vi "measure_j-t.vi"(4 "Skip pixel?":bool, 5 "Date array":string[](array[string]), 6 "Scan settings":T1={"J-V scan"=TRUE, "Start voltage (V)"=0.0, "End voltage (V)"=0.0, "Step voltage (V)"=1.4, "Scan both directions"=TRUE, "Inverted device structure"=FALSE, "Measurement delay (ms)"=10.0, "Measurement speed"=0, "Scan rate (V/s)"=0.0, "Stabilisation time (s)"=0.0, "Stabilisation mode"=0, "Stabilisation value (V or A) "=1.0, "Illumination"=0, "Stabilisation in the dark?"=FALSE, "Repeat light scans"=FALSE, "No. of repeat scans"=0.0, "Only repeat for best pixel"=1, "J-t scan"=FALSE, "J-t best pixel only"=7, "J-t start voltage (V)"=0.0, "J-t end voltage (V)"=1.4, "J-t step voltage (V)"=0.01, "Step time (s)"=0.7, "J-t scan both directions"=TRUE, "J-t inverted device structure"=FALSE, "J-t settling delay (s)"=0.0, "J-t measurement speed"=0, "J-t illumination"=2, "Max. power stabilisation"=FALSE, "Max power best pixel only"=1, "Max. power point tracker"=FALSE, "Vmp from J-V scan"=FALSE, "Max P stab. Specific voltage"=FALSE, "Vmp (V)"=1.0, "Stabilisation time step (s)"=1.0, "Total stabilisation time (s)"=100.0} {"J-t settling delay (s)" min=10.0; "J-t illumination" items=["Light only", "Dark only", "Light then dark", "Dark then light"]; "Measurement speed" items=["Fast", "Normal", "High accuracy"]; "Illumination" items=["Light only", "Dark only", "Light then dark", "Dark then light"]; "Only repeat for best pixel" items=["only for best pixel", "for best 2 pixels", "for best 3 pixels", "for best 4 pixels", "for best 5 pixels", "for best 6 pixels", "for best 7 pixels", "for all pixels"]; "No. of repeat scans" min=1.0 step=1.0; "Max power best pixel only" items=["only the best pixel", "the best 2 pixels", "the best 3 pixels", "the best 4 pixels", "the best 5 pixels", "the best 6 pixels", "the best 7 pixels", "all pixels"]; "J-t best pixel only" items=["only the best pixel", "the best 2 pixels", "the best 3 pixels", "the best 4 pixels", "the best 5 pixels", "the best 6 pixels", "the best 7 pixels", "all pixels"]; "J-t measurement speed" items=["Fast", "Normal", "High Accuracy"]; "Stabilisation mode" items=["V", "I"]; "Measurement delay (ms)" min=10.0}, 7 "Cell details cluster":T2={"Cell Position"=16, "Cell Label"="", "Pixel to measure"=0, "Area (cm^2)"=0.126, "Variable"="", "Variable value"="", "Scan settings in queue"=0, "Light or dark"="", "Measurement Type"=""} {"Pixel to measure" items=["All", "1", "2", "3", "4", "5", "6", "7", "8"]}, 8 "VISA resource name":refnum<visa-resource-name>="GPIB1::24::INSTR", 9 "Intensity (no. of suns)":string, 10 "Experiment Title":string, 11 "User Name":string) -> (3 "Jt Curve":cluster{"Y":dbl[], "Y":dbl[]}[](graph) caption="JV Curve")   [LabVIEW 2016]
uses:
  TypeDefs/scan_settings.ctl
  <vilib>/Utility/file.llb/Read Delimited Spreadsheet (DBL).vi
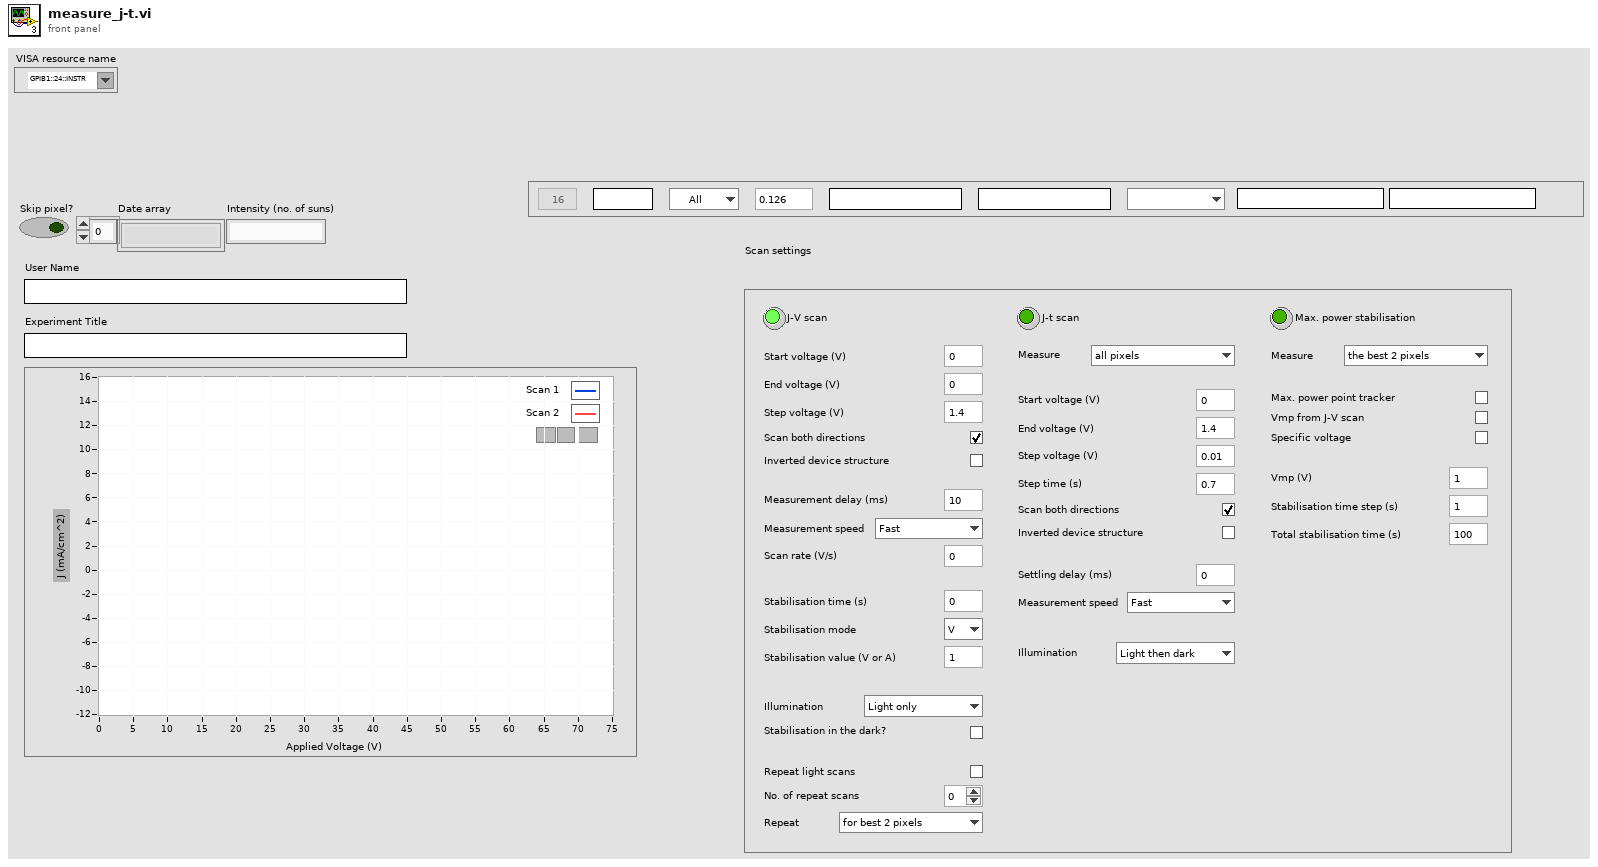
[diagram p1: front panel]
types:
  T1 = typedef "scan_settings.ctl" = cluster{"J-V scan":bool, "Start voltage (V)":dbl, "End voltage (V)":dbl, "Step voltage (V)":dbl, "Scan both directions":bool, "Inverted device structure":bool, "Measurement delay (ms)":dbl, "Measurement speed":u8, "Scan rate (V/s)":dbl, "Stabilisation time (s)":dbl, "Stabilisation mode":u16, "Stabilisation value (V or A) ":dbl, "Illumination":u16, "Stabilisation in the dark?":bool, "Repeat light scans":bool, "No. of repeat scans":dbl, "Only repeat for best pixel":u16, "J-t scan":bool, "J-t best pixel only":u16, "J-t start voltage (V)":dbl, "J-t end voltage (V)":dbl, "J-t step voltage (V)":dbl, "Step time (s)":dbl, "J-t scan both directions":bool, "J-t inverted device structure":bool, "J-t settling delay (s)":dbl, "J-t measurement speed":u16, "J-t illumination":u16, "Max. power stabilisation":bool, "Max power best pixel only":u16, "Max. power point tracker":bool, "Vmp from J-V scan":bool, "Max P stab. Specific voltage":bool, "Vmp (V)":dbl, "Stabilisation time step (s)":dbl, "Total stabilisation time (s)":dbl}
  T2 = cluster{"Cell Position":i32, "Cell Label":string, "Pixel to measure":u16, "Area (cm^2)":dbl, "Variable":string, "Variable value":string, "Scan settings in queue":u16, "Light or dark":string, "Measurement Type":string}
  T3 = typedef "imagedata.ctl" = cluster{"image type":i32, "image depth":i32, "image":u8[], "mask":u8[], "colors":u32[], "Rectangle":cluster{"left":i16, "top":i16, "right":i16, "bottom":i16}}
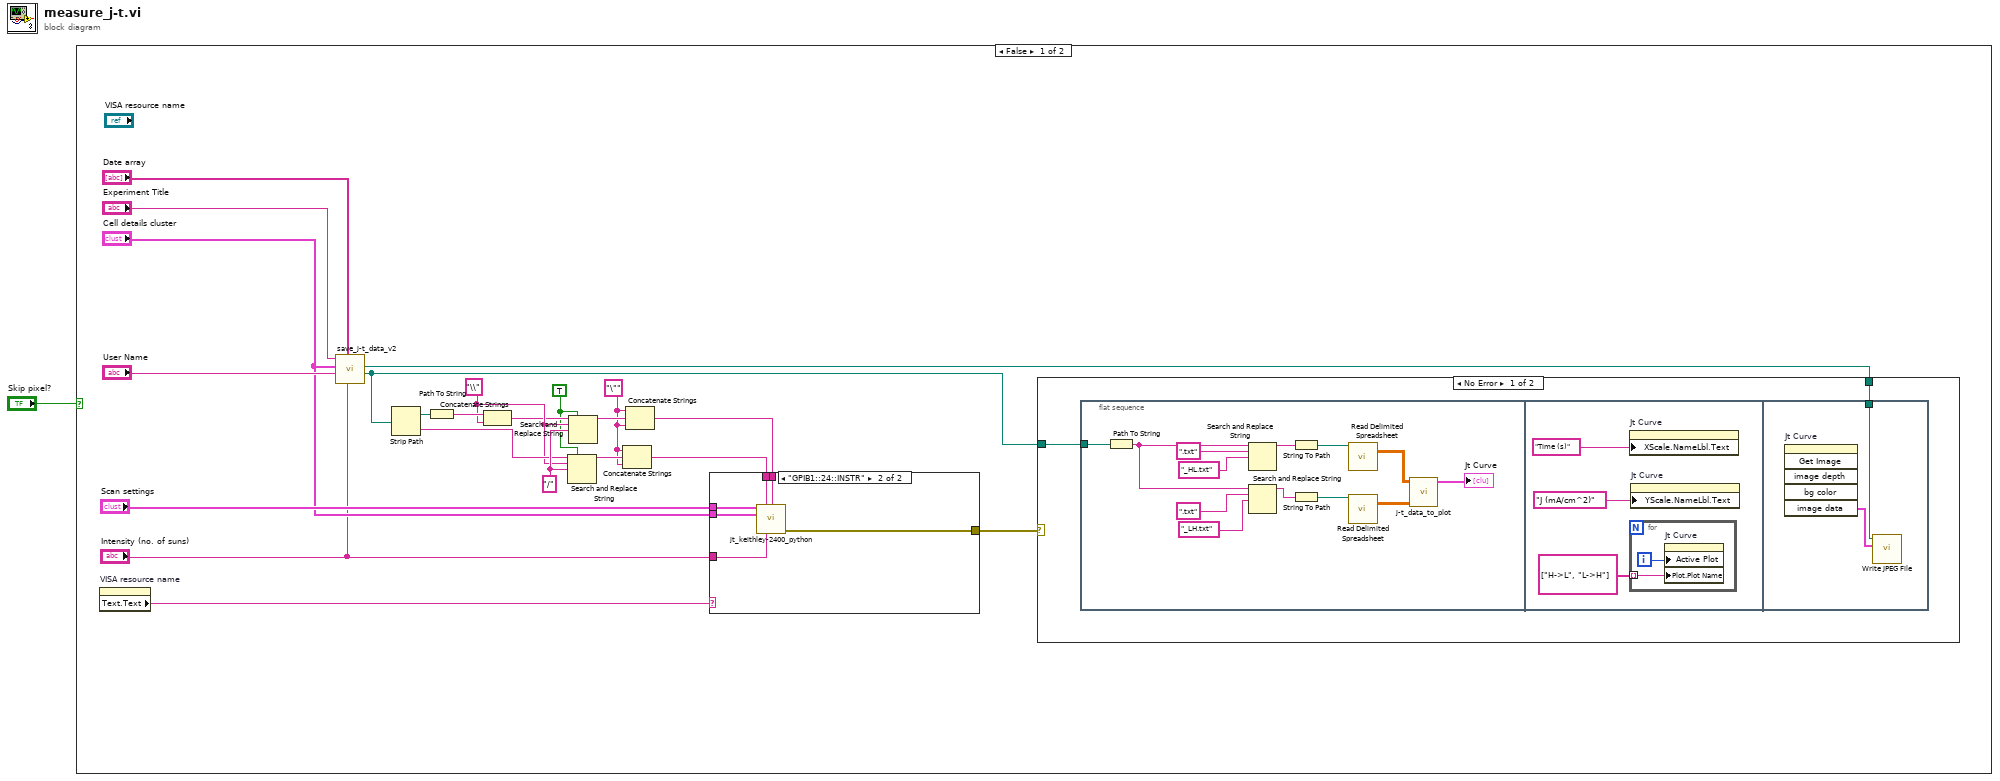
[diagram p0: block diagram]
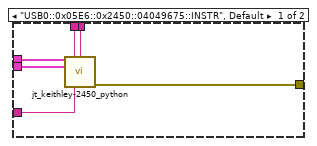
[diagram p3: hidden frame]
diagram:
  n1 = case shown="False" "Skip pixel?" {
    frame False {
      w14 = "\"" ("string")
      w11 = TRUE ("replace all? (F)")
      w19 = "/" ("search string")
      w13 = "\\" ("search string")
      n2 = property on="VISA resource name" class="VISAName"() -> ("Text.Text"=w5:string)  [unwired: 2 in, 2 out]
      n3 = call "save_j-t_data_v2.vi"("Intensity (no. of suns)"="Intensity (no. of suns)", "Date array"="Date array", "User name"="User Name", "Cell details cluster"="Cell details cluster", "Experiment title"="Experiment Title") -> ("File path for JV data"=w4:path, "File path for JV image"=w3:path)  [unwired: 3 in]
      n4 = Strip Path(path=w4) -> (stripped path=w16:path, name=w17:string)
      n5 = Path To String(path=w16) -> (string=w15:string)
      n6 = Concatenate Strings(w15, w13) -> (w12:string)
      n7 = Search and Replace String(replace all?=w11, input string=w17, search string=w13, replace string=w19) -> (result string=w18:string)  [unwired: 4 in, 3 out]
      n8 = Search and Replace String(replace all?=w11, input string=w12, search string=w13, replace string=w19) -> (result string=w20:string)  [unwired: 4 in, 3 out]
      n9 = Concatenate Strings(w14, w18, w14) -> (w9:string)
      n10 = Concatenate Strings(w14, w20, w14) -> (w10:string)
      n11 = case shown="\"GPIB1::24::INSTR\"" w5 {
        tunnel: w10 -> [w49 w57]
        tunnel: w9 -> [w50 w56]
        tunnel: "Scan settings" -> [w51 w55]
        tunnel: "Cell details cluster" -> [w48 w54]
        tunnel: "Intensity (no. of suns)" -> [w47 w53]
        tunnel: [w46 w52] -> w2
        frame "USB0::0x05E6::0x2450::04049675::INSTR", Default {
          n12 = call "jt_keithley-2450_python.vi"("Scan settings"=w51, "file name"=w50, "folder path"=w49, "Cell details cluster"=w48, "illumination intensity (suns equiv.)"=w47) -> ("error out"=w46:errorcluster)  [unwired: 10 in]
        }
        frame "GPIB1::24::INSTR" {
          n13 = call "jt_keithley-2400_python.vi"("Scan settings"=w55, "file name"=w56, "folder path"=w57, "Cell details cluster"=w54, "illumination intensity (suns equiv.)"=w53) -> ("error out"=w52:errorcluster)  [unwired: 10 in]
        }
      }
      n14 = case shown="No Error" w2 {
        tunnel: w4 -> [w25 _]
        tunnel: w3 -> [w24 _]
        frame No Error {
          n15 = flat-sequence {
            tunnel: w25 -> [w37]
            tunnel: w24 -> [w44]
            frame #0 {
              n16 = Path To String(path=w37) -> (string=w33:string)
              n17 = Search and Replace String(input string=w33, search string=".txt", replace string="_HL.txt" ("replace string (\"\")")) -> (result string=w36:string)  [unwired: 5 in, 3 out]
              n18 = Search and Replace String(input string=w33, search string=".txt", replace string="_LH.txt" ("replace string (\"\")")) -> (result string=w28:string)  [unwired: 5 in, 3 out]
              n19 = String To Path(string=w36) -> (path=w35:path)
              n20 = String To Path(string=w28) -> (path=w27:path)
              n21 = call-poly <vilib>:"Read Delimited Spreadsheet.vi"("file path (dialog if empty)"=w35) -> ("all rows"=w34:dbl[][])  [unwired: 9 in, 5 out]
              n22 = call-poly <vilib>:"Read Delimited Spreadsheet.vi"("file path (dialog if empty)"=w27) -> ("all rows"=w26:dbl[][])  [unwired: 9 in, 5 out]
              n23 = call "j-t_data_to_plot.vi"("Data Array 2"=w26, "Data Array"=w34) -> ("JV Curve"=→"Jt Curve":cluster{"Y":dbl[], "Y":dbl[]}[])  [unwired: 9 in]
            }
            frame #1 {
              n24 = property on="Jt Curve" class="XYGraph (strict)"("XScale.NameLbl.Text"="Time (s)" ("Y Scale.Name Label.Text")) -> ()  [unwired: 2 in, 2 out]
              n25 = for {
                tunnel: string[] ["H->L", "L->H"] ("Measurement queue") -> [w42] mode=indexing
                i -> [w43]
                n26 = property on="Jt Curve" class="XYGraph (strict)"("Active Plot"=w43, "Plot.Plot Name"=w42) -> ()  [unwired: 2 in, 2 out]
              }
              n27 = property on="Jt Curve" class="XYGraph (strict)"("YScale.NameLbl.Text"="J (mA/cm^2)" ("Y Scale.Name Label.Text")) -> ()  [unwired: 2 in, 2 out]
            }
            frame #2 {
              n28 = invoke on="Jt Curve" class="XYGraph (strict)" method="Get Image"() -> ("image data"=w45:T3)  [unwired: 6 in, 5 out]
              n29 = call <vilib>:"Write JPEG File.vi"("image data"=w45, "path to JPEG file"=w44) -> ()  [unwired: 8 in, 2 out]
            }
          }
        }
        frame Error {
        }
      }
    }
    frame True {
    }
  }
